vi "SubVI_Save_Calibration_Data_rev2.vi"(8 "error in (no error)":errorcluster, 11 "Channel in":T1) -> (0 "error out":errorcluster)   [LabVIEW 2020]
uses:
  <extravilib>/ChannelInstances/Stream-a[.](dbl)/)Channel.ctl
  <extravilib>/ChannelInstances/Stream-a[.](dbl)/EndpointRead.vi
  Global 1.vi
  <extravilib>/ChannelInstances/Stream-a[.](dbl)/)Channel.vi
  <resource>/ChannelSupport/_ChannelSupport/WaitIfNeeded.vi
  <extravilib>/ChannelInstances/Stream-a[.](dbl).lvlib
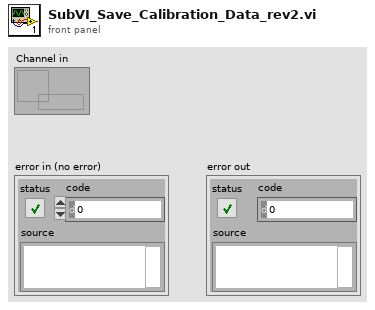
[diagram p1: front panel]
types:
  T1 = typedef "Stream-a[.](dbl).lvlib/)Channel.ctl" = refnum<queue>
  T2 = enum16{"open", "open or create", "create or replace", "create", "open (read-only)"}
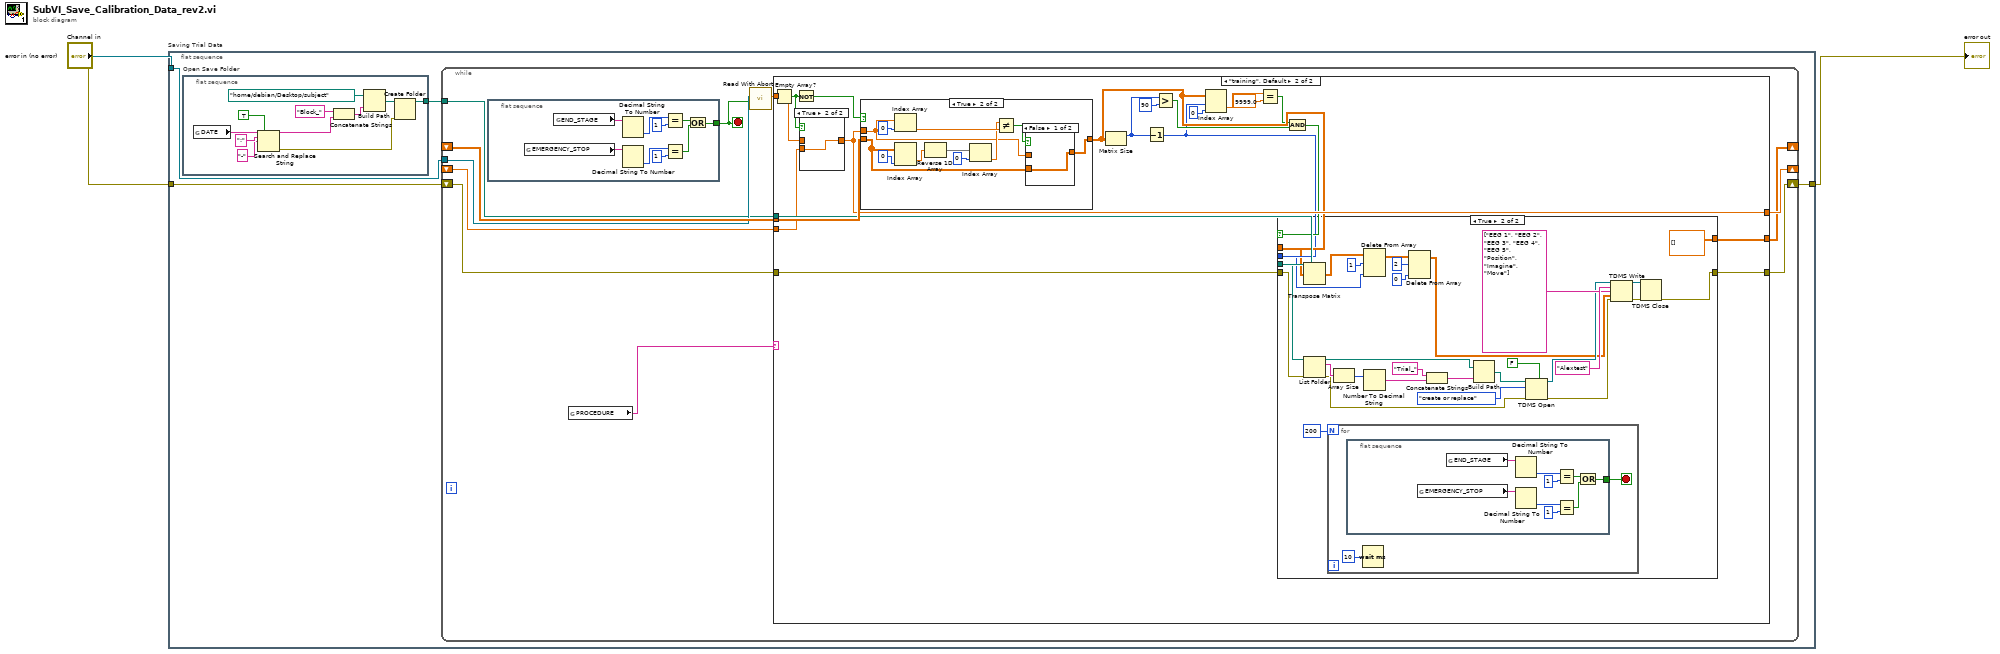
[diagram p0: block diagram]
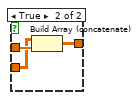
[diagram p6: hidden frame]
diagram:
  n1 = flat-sequence "Saving Trial Data" {
    tunnel: "Channel in" -> [w6]
    tunnel: [w5] -> w2
    tunnel: "error in (no error)" -> [w4]
    frame #0 {
      n2 = flat-sequence "Open Save Folder" {
        tunnel: [w14] -> w7
        frame #0 {
          n3 = global read "Global 1.vi" "DATE"() -> (w8:string)
          n4 = Search and Replace String(replace all?=TRUE ("replace all? (F)"), input string=w8, search string=":" ("input string"), replace string="-" ("replace string (\"\")")) -> (result string=w11:string, error out=w10:errorcluster)  [unwired: 4 in, 2 out]
          n5 = Concatenate Strings("Block_" ("string"), w11) -> (w15:string)
          n6 = Build Path(base path=path "/home/debian/Desktop/subject", name or relative path=w15) -> (appended path=w17:path)
          n7 = Create Folder(path (use dialog)=w17, error in=w10) -> (created path=w14:path)  [unwired: 1 in, 2 out]
        }
      }
      n8 = while {
        shift-right: [w20] -> _
        shift-left: _ -> [w29]
        tunnel: w6 -> [w28]
        shift-right: [w26] -> w5
        shift-left: w4 -> [w27]
        tunnel: w7 -> [w25]
        shift-right: [w22] -> _
        shift-left: _ -> [w23]
        stop <- w21 stop-if-true
        n9 = flat-sequence {
          tunnel: [w113] -> w21
          frame #0 {
            n10 = global read "Global 1.vi" "EMERGENCY_STOP"() -> (w116:string)
            n11 = global read "Global 1.vi" "END_STAGE"() -> (w121:string)
            n12 = Decimal String To Number(string=w121) -> (number=w120:i32)  [unwired: 2 in, 1 out]
            n13 = Decimal String To Number(string=w116) -> (number=w118:i32)  [unwired: 2 in, 1 out]
            n14 = Equal?(x=w120, y=1) -> (x = y?=w114:bool)
            n15 = Equal?(x=w118, y=1) -> (x = y?=w115:bool)
            n16 = Or(x=w114, y=w115) -> (x .or. y?=w113:bool)
          }
        }
        n17 = global read "Global 1.vi" "PROCEDURE"() -> (w19:string)
        n18 = call <extravilib>:"Read With Abort.vi"("abort"=w21, "channel"=w28) -> ("element"=w24:dbl[])  [unwired: 4 in, 5 out]
        n19 = case shown="\"training\", Default" w19 {
          tunnel: w29 -> [w31 w52]
          tunnel: w27 -> [w30 w51]
          tunnel: [w30 w50] -> w26
          tunnel: w25 -> [_ w49]
          tunnel: w24 -> [_ w48]
          tunnel: w23 -> [w32 w47]
          tunnel: [w32 w46] -> w22
          tunnel: [w31 w36] -> w20
          frame "tutorial" {
          }
          frame "training", Default {
            n20 = Empty Array?(array=w48) -> (empty?=w34:bool)
            n21 = Not(x=w34) -> (.not. x?=w33:bool)
            n22 = case shown="True" w34 {
              tunnel: w48 -> [w95 _]
              tunnel: [w95 w96] -> w46
              tunnel: w47 -> [_ w96]
              frame False {
              }
              frame True {
              }
            }
            n23 = case shown="True" w33 {
              tunnel: w52 -> [w97 w100]
              tunnel: w46 -> [_ w98]
              tunnel: [w97 w108] -> w44
              frame False {
              }
              frame True {
                n24 = Index Array(array=w98, index=0) -> (element=w106:dbl)
                n25 = Index Array(array=w100, index (col)=0 ("disabled index (row)")) -> (element=w103:dbl[])  [unwired: 1 in]
                n26 = Reverse 1D Array(array=w103) -> (reversed array=w104:dbl[])
                n27 = Index Array(array=w104, index=0 ("disabled index (row)")) -> (element=w102:dbl)
                n28 = Not Equal?(x=w102, y=w106) -> (x != y?=w99:bool)
                n29 = case shown="False" w99 {
                  tunnel: [w109 w112] -> w108
                  tunnel: w98 -> [_ w111]
                  tunnel: w100 -> [w109 w110]
                  frame False {
                  }
                  frame True {
                    n30 = Build Array (concatenate)(w110, w111) -> (w112:dbl[][])
                  }
                }
              }
            }
            n31 = Matrix Size(0:w44) -> (1:w43:i32)  [unwired: 1 out]
            n32 = Decrement(x=w43) -> (x-1=w35:i32)
            n33 = Greater?(x=w43, y=90) -> (0:w38:bool)
            n34 = Index Array(array=w44, index (row)=w35, index (col)=0 ("disabled index (col)")) -> (element=w41:dbl)
            n35 = Equal?(x=w41, y=9999.0) -> (x = y?=w39:bool)
            n36 = And(x=w39, y=w38) -> (x .and. y?=w37:bool)
            n37 = case shown="True" w37 {
              tunnel: w44 -> [w53 w65]
              tunnel: w51 -> [w54 w67]
              tunnel: [w54 w66] -> w50
              tunnel: w49 -> [_ w68]
              tunnel: [w53 dbl[][] []] -> w36
              tunnel: w35 -> [_ w58]
              frame False {
              }
              frame True {
                n38 = Transpose Matrix(1:w65) -> (0:w57:dbl[][])
                n39 = List Folder(path=w68, error in=w67) -> (path out=w64:path, filenames=w73:string[], error out=w71:errorcluster)  [unwired: 2 in, 1 out]
                n40 = for {
                  N: u32 200 ("milliseconds to wait") -> [_]
                  stop <- w84 stop-if-true
                  n41 = flat-sequence {
                    tunnel: [w86] -> w84
                    frame #0 {
                      n42 = global read "Global 1.vi" "EMERGENCY_STOP"() -> (w89:string)
                      n43 = global read "Global 1.vi" "END_STAGE"() -> (w94:string)
                      n44 = Decimal String To Number(string=w94) -> (number=w93:i32)  [unwired: 2 in, 1 out]
                      n45 = Decimal String To Number(string=w89) -> (number=w91:i32)  [unwired: 2 in, 1 out]
                      n46 = Equal?(x=w93, y=1) -> (x = y?=w87:bool)
                      n47 = Equal?(x=w91, y=1) -> (x = y?=w88:bool)
                      n48 = Or(x=w87, y=w88) -> (x .or. y?=w86:bool)
                    }
                  }
                  n49 = Wait (ms)(milliseconds to wait=u32 10) -> ()  [unwired: 1 out]
                }
                n50 = Array Size(array=w73) -> (size(s)=w74:i32)
                n51 = Delete From Array(array=w57, length=1, index (col)=w58) -> (array with subset deleted=w56:dbl[][])  [unwired: 1 in, 1 out]
                n52 = Number To Decimal String(number=w74) -> (decimal integer string=w72:string)  [unwired: 1 in]
                n53 = Delete From Array(array=w56, length=2, index (col)=0 ("disabled index (col)")) -> (array with subset deleted=w61:dbl[][])  [unwired: 1 in, 1 out]
                n54 = Concatenate Strings("Trial_" ("string"), w72) -> (w83:string)
                n55 = Build Path(base path=w64, name or relative path=w83) -> (appended path=w81:path)
                n56 = TDMS Open(5:FALSE ("create index file? (T)"), 8:w71, 10:T2."create or replace" ("operation (0:open)"), 11:w81) -> (0:w70:errorcluster, 3:w77:refnum<k34>)  [unwired: 3 in]
                n57 = TDMS Write(0:w77, 5:"Alextest" ("group name in (Untitled)"), 7:string[] ["EEG 1", "EEG 2", "EEG 3", "EEG 4", "EEG 5", "Position", "Imagine", "Move"] ("channel name(s) in (Untitled)"), 9:w61, 11:w70) -> (4:w80:refnum<k34>, 15:w69:errorcluster)  [unwired: 1 in, 2 out]
                n58 = TDMS Close(8:w69, 11:w80) -> (0:w66:errorcluster)  [unwired: 1 out]
              }
            }
          }
        }
      }
    }
  }
  "error out" <- w2
